vi "LS336monitor.vi"(1 "Output 2":u16(ring) items=["A", "B", "C", "D"], 2 "Output 1":u16(ring) items=["A", "B", "C", "D"]) -> (0 "VISA resource name 2":refnum<visa-resource-name>)   [LabVIEW 2024]
panel:
  in  "OK Button":bool
  in  "VISA resource name":refnum<visa-resource-name>
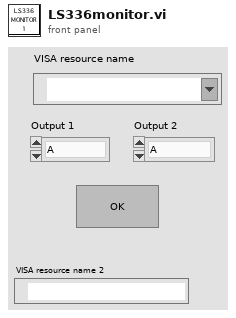
[diagram p1: front panel]
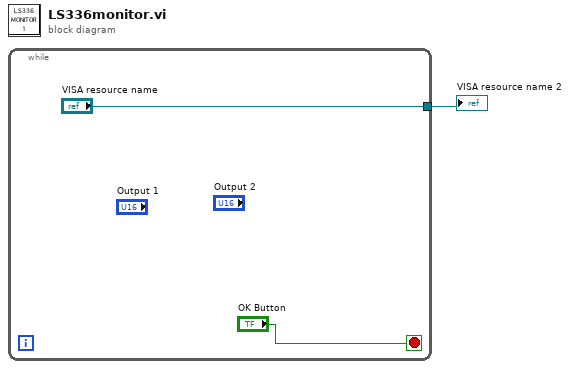
[diagram p0: block diagram]
diagram:
  n1 = while {
    tunnel: ["VISA resource name"] -> w1
    stop <- "OK Button" stop-if-true
  }
  "VISA resource name 2" <- w1
